vi "Process Container.vi"() -> ()   [LabVIEW 2013, in "Caraya.lvlib" / "Basic Test Manager.lvclass"]
uses:
  Basic Test Manager.lvclass
  Test Result/Test Event Data.ctl
  Test Result/Test Result.lvclass
panel:
  out "error":errorcluster
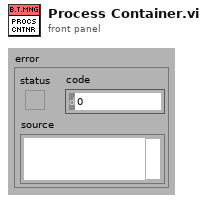
[diagram p1: front panel]
types:
  T1 = typedef "Caraya.lvlib/Test Result.lvclass/Test Event Data.ctl" = cluster{"Label":string, "Argument":variant}
  T2 = typedef "Caraya.lvlib/Test Result.lvclass/Test Event.ctl" = refnum<user-event>
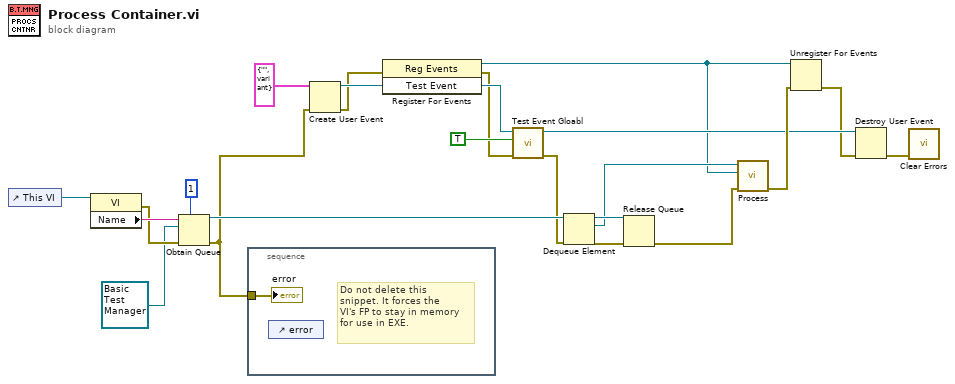
[diagram p0: block diagram]
diagram:
  n1 = control-ref of="This VI"() -> (w22:refnum<vi>)
  n2 = property class="VI"(reference=w22) -> (error out=w20:errorcluster, "Name"=w21:string)  [unwired: 1 in, 1 out]
  n3 = Obtain Queue(max queue size (-1, unlimited)=1, name (unnamed)=w21, element data type=refnum<class "Basic Test Manager.lvclass"> refnum ("element"), error in (no error)=w20) -> (queue out=w17:refnum<queue>, error out=w9:errorcluster)  [unwired: 1 in, 1 out]
  n4 = stacked-sequence {
    tunnel: w9 -> [w23]
    frame #0 {
      # "Do not delete this\nsnippet. It forces the\nVI's FP to stay in memory\nfor use in EXE."
      n5 = control-ref of="error"() -> ()  [unwired: 1 out]
      "error" <- w23
    }
  }
  n6 = Create User Event(user event datatype=T1 {"Label"="", "Argument"=variant} ("Test Event"), error in=w9) -> (user event=w8:refnum<user-event>, error out=w7:errorcluster)
  n7 = register-events(error in=w7, w8) -> (reference out=w1:refnum<event-registration>, error out=w6:errorcluster)  [unwired: 1 in]
  n8 = call "Test Event Gloabl.vi"("error in (no error)"=w6, "Set (F)"=TRUE, "Test Event in"=w8) -> ("error out"=w11:errorcluster, "Test Event out"=w4:T2)  [unwired: 5 in, 2 out]
  n9 = Dequeue Element(queue=w17, error in (no error)=w11) -> (queue out=w16:refnum<queue>, element=w14:refnum<class "Basic Test Manager.lvclass">, error out=w15:errorcluster)  [unwired: 1 in, 1 out]
  n10 = Release Queue(queue=w16, error in (no error)=w15) -> (error out=w13:errorcluster)  [unwired: 1 in, 2 out]
  n11 = call "Process.vi"("error in (no error)"=w13, "Event Registration Refnum"=w1, "Test Manager in"=w14) -> ("error out"=w5:errorcluster)  [unwired: 7 in, 1 out]
  n12 = Unregister For Events(event registration refnum=w1, error in=w5) -> (error out=w3:errorcluster)
  n13 = Destroy User Event(user event=w4, error in=w3) -> (error out=w2:errorcluster)
  n14 = call <vilib>:"Clear Errors.vi"("error in (no error)"=w2) -> ()  [unwired: 6 in, 1 out]
